vi "Spawn.vi"(7 "Actor in":refnum<class "Actor.lvclass">, 9 "UID":string, 10 "Actor":refnum<class "Actor.lvclass">) -> (0 "Error out":errorcluster, 5 "Actor out":refnum<class "Actor.lvclass">)   [LabVIEW 2025, in "jettl.lvlib" / "Actor.lvlib"]
uses:
  Actor.lvlib
  Actor/Actor.lvclass
  Error/Error.lvlib
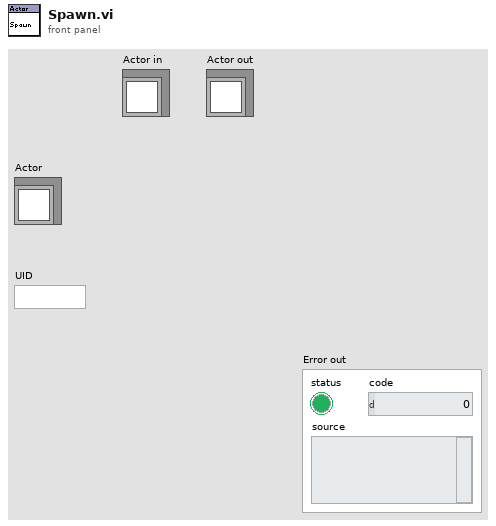
[diagram p1: front panel]
types:
  T1 = typedef "jettl.lvlib/Actor.lvlib/Child UIDs.ctl" = set{string}
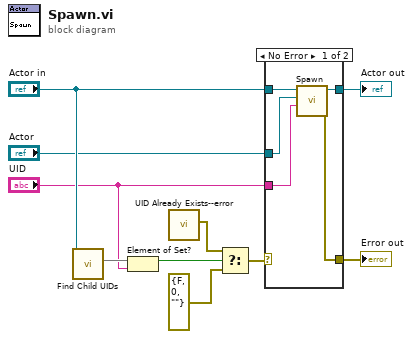
[diagram p0: block diagram]
diagram:
  n1 = call-dynamic "Find Child UIDs.vi"("Actor in"="Actor in") -> ("Child UIDs"=w8:T1)  [unwired: 10 in]
  n2 = Element of Set?(10:"UID", 11:w8) -> (3:w4:bool)
  n3 = call "UID Already Exists--error.vi"() -> ("Error"=w5:errorcluster)  [unwired: 11 in]
  n4 = Select(t=w5, s=w4, f=errorcluster {"status"=FALSE, "code"=0, "source"=""}) -> (s? t:f=w2:errorcluster)
  n5 = case shown="No Error" w2 {
    selector: w2 -> [_ w16]
    tunnel: "UID" -> [w11 _]
    tunnel: "Actor in" -> [w13 w17]
    tunnel: [w15 w16] -> w10
    tunnel: [w14 w17] -> w9
    tunnel: "Actor" -> [w12 _]
    frame No Error {
      n6 = call-dynamic "Spawn.vi"("UID"=w11, "Actor"=w12, "Actor in"=w13) -> ("Error out"=w15:errorcluster, "Actor out"=w14:refnum<class "Actor.lvclass">)  [unwired: 7 in]
    }
    frame Error {
    }
  }
  "Error out" <- w10
  "Actor out" <- w9
